vi "timer.vi"(10 "Time":dbl, 11 "Set":bool) -> (3 "Out":bool)   [LabVIEW 2013]
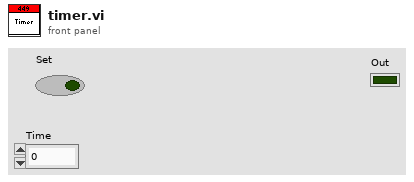
[diagram p1: front panel]
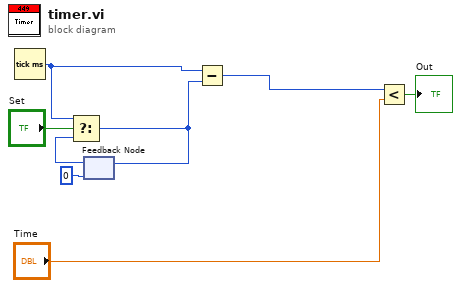
[diagram p0: block diagram]
diagram:
  n1 = Tick Count (ms)() -> (millisecond timer value=w1:u32)
  n2 = feedback #1(u32 0 ("millisecond timer value")) -> (w8:u32)
  n3 = Select(t=w1, s="Set", f=w8) -> (s? t:f=w5:u32)
  n4 = feedback-in #1(w5) -> ()
  n5 = Subtract(x=w1, y=w5) -> (x-y=w4:u32)
  n6 = Less?(x=w4, y="Time") -> (x < y?=→"Out":bool)
